vi "Calibrate Adjust Sense.vi"(8 "error in (no error)":errorcluster, 10 "Sense Value":dbl format="%#_6e", 11 "VISA resource name":refnum<visa-resource-name>) -> (0 "error out":errorcluster, 3 "VISA resource name out":refnum<visa-resource-name>)   [LabVIEW 2020, in "Keithley 2450.lvlib"]
doc: "Calibrates the sense function/range currently configured with the given characterized Sense Value."
uses:
  <instrlib>/Keithley 2450/Keithley 2450.lvlib
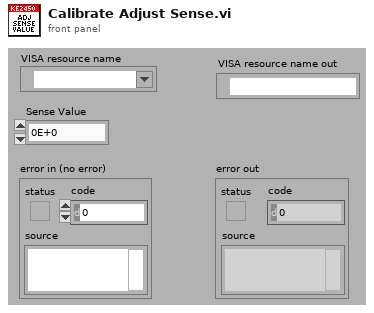
[diagram p1: front panel]
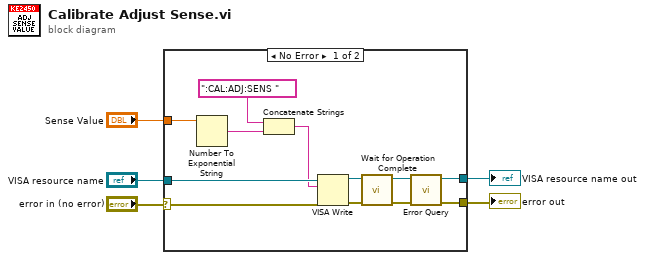
[diagram p0: block diagram]
diagram:
  n1 = case shown="No Error" "error in (no error)" {
    selector: "error in (no error)" -> [w17 w19]
    tunnel: [w7 w19] -> w4
    tunnel: "VISA resource name" -> [w16 w18]
    tunnel: [w6 w18] -> w2
    tunnel: "Sense Value" -> [w12 _]
    frame No Error {
      n2 = Number To Exponential String(number=w12) -> (E-format string=w13:string)  [unwired: 3 out]
      n3 = Concatenate Strings(":CAL:ADJ:SENS " ("string"), w13) -> (w14:string)
      n4 = VISA Write(VISA resource name=w16, write buffer=w14, error in (no error)=w17) -> (VISA resource name out=w10:refnum<visa-resource-name>, error out=w11:errorcluster)  [unwired: 1 out]
      n5 = call <instrlib>:"Wait for Operation Complete.vi"("error in (no error)"=w11, "VISA resource name"=w10) -> ("error out"=w8:errorcluster, "VISA resource name out"=w9:refnum<visa-resource-name>)  [unwired: 8 in]
      n6 = call <instrlib>:"Error Query.vi"("error in (no error)"=w8, "VISA resource name"=w9) -> ("error out"=w7:errorcluster, "VISA resource name out"=w6:refnum<visa-resource-name>)  [unwired: 6 in, 2 out]
    }
    frame Error {
      # "Do nothing if error condition"
    }
  }
  "error out" <- w4
  "VISA resource name out" <- w2
